vi "HW_Gantner_Construct Initial Modu Configuration.vi"(7 "SampleRate":dbl, 8 "error in":errorcluster, 9 "Modu[] in":T2[](array[typedef]), 10 "ModCFG in":T1[](array[typedef]), 11 "CHdef":path) -> (0 "error out":errorcluster, 2 "ModCFG to File":T1[](array[typedef]), 3 "ModuInSysCFG":T1[](array[typedef]))   [LabVIEW 2016]
uses:
  Gantner Device Info.ctl
  Ctrls/HardWare _ Module Configuration.ctl
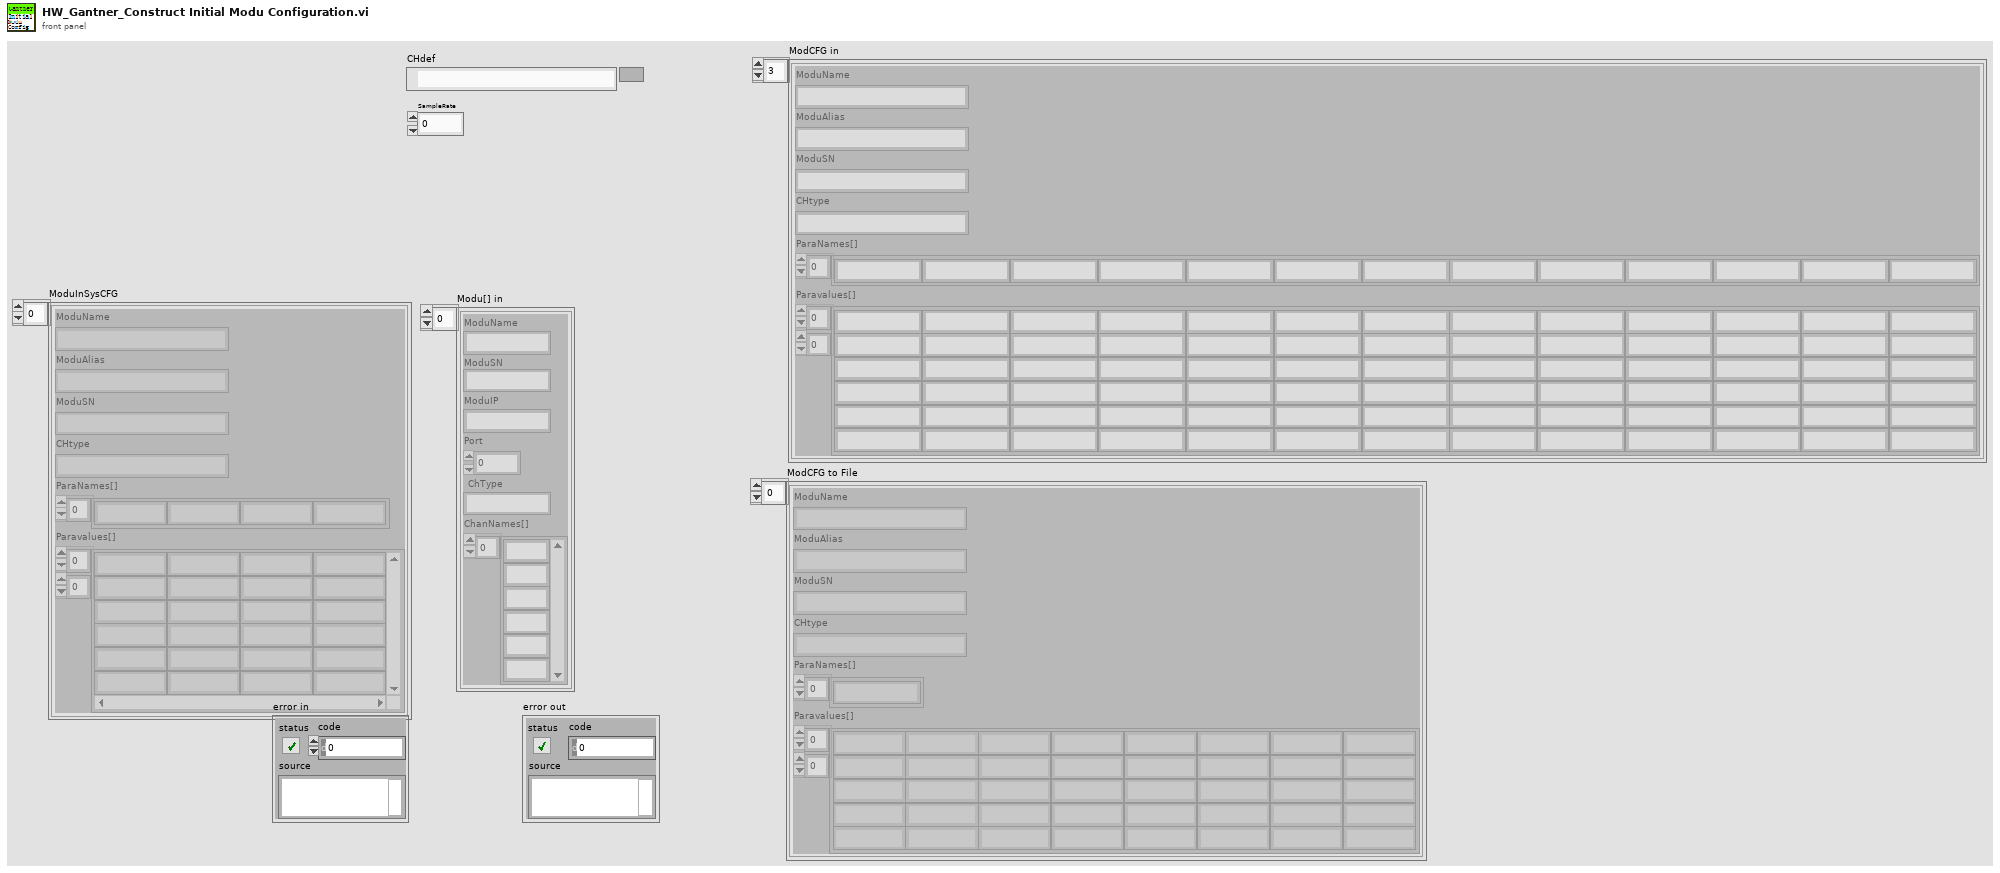
[diagram p1: front panel]
types:
  T1 = typedef "HardWare _ Module Configuration.ctl" = cluster{"ModuName":string, "ModuAlias":string, "ModuSN":string, "CHtype":string, "ParaNames[]":string[], "Paravalues[]":string[][]}
  T2 = typedef "Gantner Device Info.ctl" = cluster{"ModuName":string, "ModuSN":string, "ModuIP":string, "Port":i32, "ChType":string, "ChanNames[]":string[]}
  T3 = typedef "HardWare _ Channel Configurations PopUp Type.ctl" = cluster{"Pop Type":T4, "PopValue":string}
  T4 = typedef "POP_Data Type.ctl" = enum16{"NO POPUP", "Unkown", "String", "Integer", "Float", "Color", "Boolean", "Ring", "Captioned String", "Captioned Integer", "Button Color", "2 Int Cluster", "4 Int Cluster", "6-Dbl Cluster", "Path", "Combox", "Time", "ShotCut String"}
  T5 = cluster{"ParaNames":string[], "DfltPara":string[], "Types":string[], "PopTypes":T3[]}
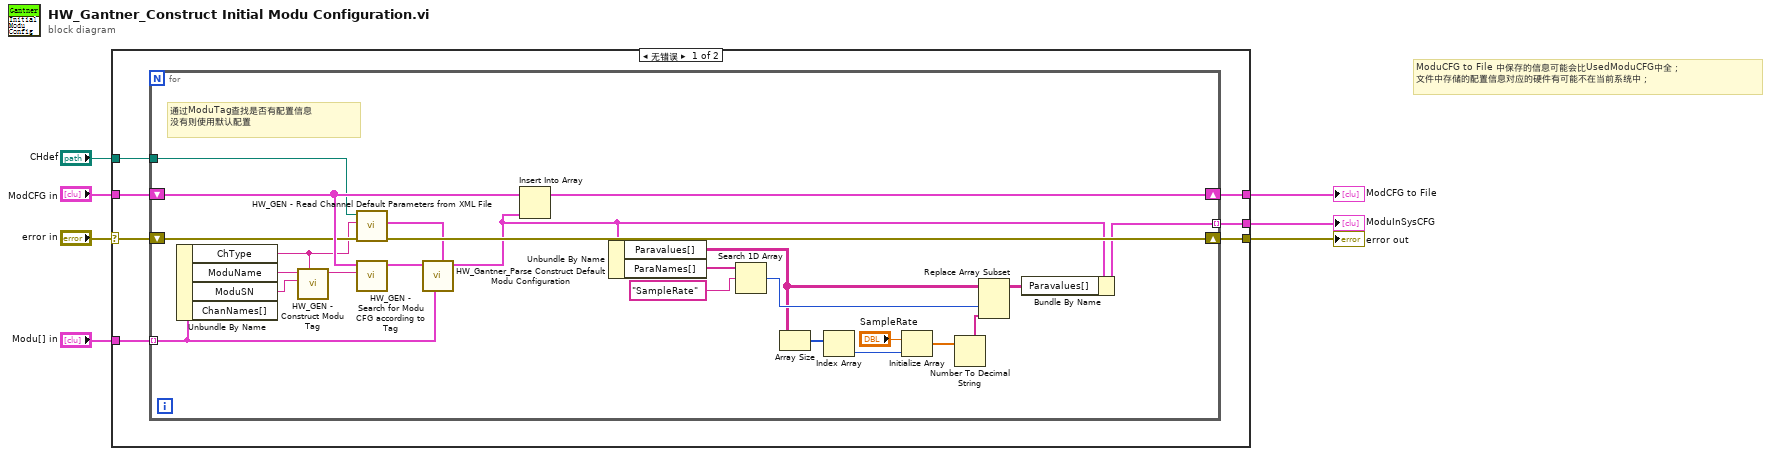
[diagram p0: block diagram]
diagram:
  # "ModuCFG to File 中保存的信息可能会比UsedModuCFG中全；\n文件中存储的配置信息对应的硬件有可能不在当前系统中；"
  n1 = case shown="无错误" "error in" {
    selector: "error in" -> [w8 w39]
    tunnel: "Modu[] in" -> [w14 _]
    tunnel: [w13 _] -> w6
    tunnel: [w12 _] -> w5
    tunnel: [w11 w39] -> w4
    tunnel: "CHdef" -> [w10 _]
    tunnel: "ModCFG in" -> [w9 _]
    frame No Error {
      n2 = for {
        shift-right: [w30] -> w11
        shift-left: w8 -> [w34]
        tunnel: w14 -> [w29] mode=indexing
        shift-right: [w31] -> w12
        shift-left: w9 -> [w36]
        tunnel: [w17] -> w13 mode=indexing
        tunnel: w10 -> [w35]
        # "通过ModuTag查找是否有配置信息\n没有则使用默认配置"
        n3 = Unbundle By Name(w29) -> ("ChType"=w28:string, "ModuName"=w33:string, "ModuSN"=w32:string)  [unwired: 1 out]
        n4 = call "HW_GEN - Construct Modu Tag.vi"("ChanType"=w28, "ModSN"=w32, "ModName"=w33) -> ("String"=w37:string)  [unwired: 8 in]
        n5 = call "HW_GEN - Read Channel Default Parameters from XML File.vi"("error in"=w34, "ChanType"=w28, "path to XML document"=w35) -> ("错误输出"=w30:errorcluster, "Chan dflt Para out"=w15:T5)  [unwired: 7 in]
        n6 = call "HW_GEN - Search for Modu CFG according to Tag.vi"("ModuTag"=w37, "ModuCFG[]"=w36) -> ("ModuCFG out"=w38:T1)  [unwired: 7 in, 2 out]
        n7 = call "HW_Gantner_Parse Construct Default Modu Configuration.vi"("Chan dflt Para in"=w15, "DevInfo"=w29, "ModuCFG from File"=w38) -> ("ModuCFG out"=w27:T1)  [unwired: 8 in]
        n8 = Insert Into Array(array=w36, new element=w27) -> (w31:T1[])  [unwired: 1 in]
        n9 = Unbundle By Name(w27) -> ("Paravalues[]"=w23:string[][], "ParaNames[]"=w26:string[])
        n10 = Search 1D Array(1D array=w26, element="SampleRate" ("元素")) -> (index of element=w24:i32)  [unwired: 1 in]
        n11 = Array Size(array=w23) -> (size(s)=w22:i32[])
        n12 = Index Array(array=w22) -> (element=w21:i32)  [unwired: 1 in]
        n13 = Initialize Array("SampleRate", w21) -> (w19:dbl[])
        n14 = Number To Decimal String(number=w19) -> (decimal integer string=w18:string[])  [unwired: 1 in]
        n15 = Replace Array Subset(array=w23, new element=w18, index (col)=w24) -> (w16:string[][])  [unwired: 1 in]
        n16 = Bundle By Name(cluster=w27, "Paravalues[]"=w16) -> (w17:T1)
      }
    }
    frame Error {
    }
  }
  "ModuInSysCFG" <- w6
  "ModCFG to File" <- w5
  "error out" <- w4
